vi "Read Measure--SubVI.vi"(8 "error in (no error)":errorcluster, 10 "Device":T9, 11 "Data Cluster":T1 {"Flexi-Flow Devices"."Control State"."Control Mode" items=["Bus/RS232"=0, "FLOW-BUS slave"=2, "Valve close"=3, "Controller idle"=4, "Setpoint 100%"=7, "Valve fully open"=8, "Calibration mode"=9, "Setpoint 0%"=12, "RS232"=18, "Valve steering"=20, "Valve safe state"=22]}) -> (0 "error out":errorcluster, 3 "Data Cluster Out":T1 {"Flexi-Flow Devices"."Control State"."Control Mode" items=["Bus/RS232"=0, "FLOW-BUS slave"=2, "Valve close"=3, "Controller idle"=4, "Setpoint 100%"=7, "Valve fully open"=8, "Calibration mode"=9, "Setpoint 0%"=12, "RS232"=18, "Valve steering"=20, "Valve safe state"=22]})   [LabVIEW 2024, in "FlexiFlowInterfaceCH2.lvlib"]
uses:
  FlexiFlowInterfaceCH2.lvlib
  FlexiFlowDevice--enum.ctl
  Module Data--cluster.ctl
  Modbus TCP Connection Settings--cluster.ctl
  Modbus Flexi-Flow State--cluster.ctl
  <vilib>/Plasmionique/MB Master/MB_Master_TCP/MB_Master_TCP.lvclass
  Device Type--enum.ctl
  Modbus Flexi-Flow Controls--cluster.ctl
  Modbus Flexi-Flow API/Control Mode--enum.ctl
  Modbus Flexi-Flow API/Control Function Values--enum.ctl
  Modbus Flexi-Flow Measure State--cluster.ctl
  Modbus Flexi-Flow API/Bronkhorst Flexi-Flow ModbusTCP API.lvlib
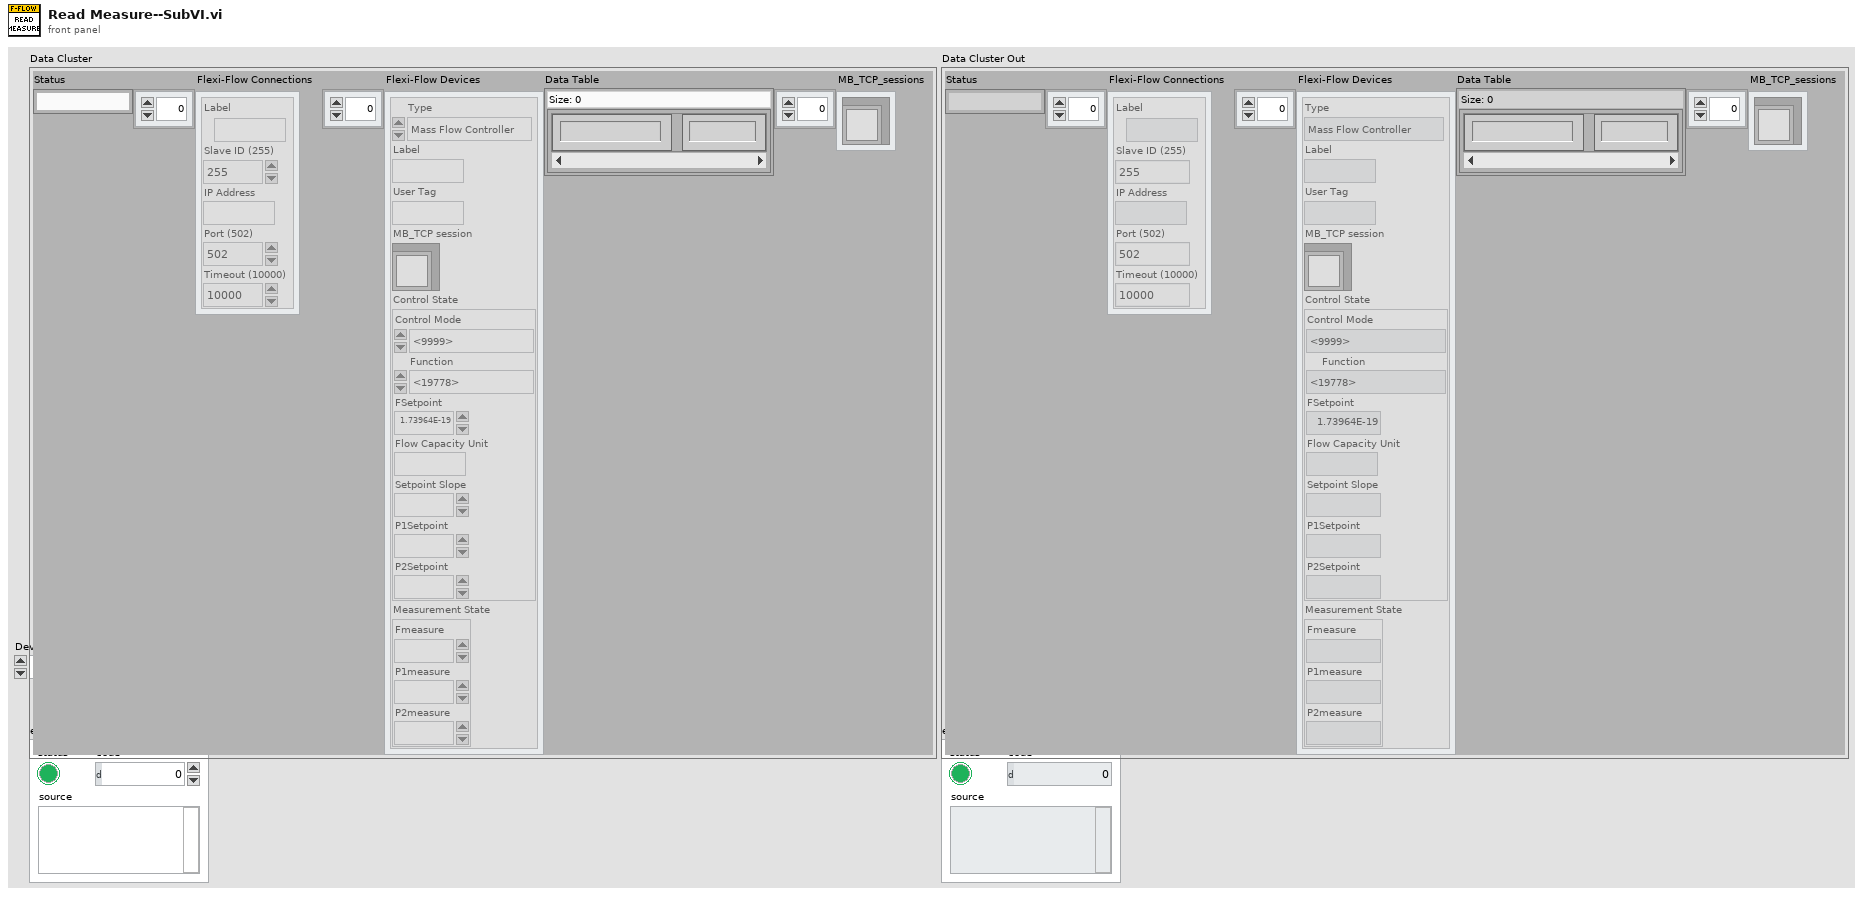
[diagram p1: front panel]
types:
  T1 = typedef "FlexiFlowInterfaceCH2.lvlib/Module Data--cluster.ctl" = cluster{"Status":string, "Flexi-Flow Connections":T2[], "Flexi-Flow Devices":T3[], "Data Table":map{string, dbl}, "MB_TCP_sessions":refnum<class "MB_Master_TCP.lvclass">[]}
  T2 = typedef "FlexiFlowInterfaceCH2.lvlib/Modbus TCP Connection Settings--cluster.ctl" = cluster{"Label":string, "Slave ID (255)":u8, "IP Address":string, "Port (502)":u16, "Timeout (10000)":i32}
  T3 = typedef "FlexiFlowInterfaceCH2.lvlib/Modbus Flexi-Flow State--cluster.ctl" = cluster{"Type":T4, "Label":string, "User Tag":string, "MB_TCP session":refnum<class "MB_Master_TCP.lvclass">, "Control State":T5, "Measurement State":T8}
  T4 = typedef "FlexiFlowInterfaceCH2.lvlib/Device Type--enum.ctl" = enum16{"Mass Flow Controller", "Mass Flow Meter"}
  T5 = typedef "FlexiFlowInterfaceCH2.lvlib/Modbus Flexi-Flow Controls--cluster.ctl" = cluster{"Control Mode":T6, "Function":T7, "FSetpoint":sgl, "Flow Capacity Unit":string, "Setpoint Slope":u16, "P1Setpoint":sgl, "P2Setpoint":sgl}
  T6 = typedef "Bronkhorst Flexi-Flow ModbusTCP API.lvlib/Control Mode--enum.ctl" = u16
  T7 = typedef "Bronkhorst Flexi-Flow ModbusTCP API.lvlib/Control Function Values--enum.ctl" = enum16{"Flow", "Upstream pressure", "Downstream pressure", "Flow with upstream pressure limit", "Flow with downstream pressure limit", "Upstream pressure with flow limit", "Downstream pressure with flow limit"}
  T8 = typedef "FlexiFlowInterfaceCH2.lvlib/Modbus Flexi-Flow Measure State--cluster.ctl" = cluster{"Fmeasure":dbl, "P1measure":sgl, "P2measure":sgl}
  T9 = typedef "FlexiFlowInterfaceCH2.lvlib/FlexiFlowDevice--enum.ctl" = enum16{"Hydrogen Inlet", "Nitrogen Inlet", "Cathode Outlet", "Anode Outlet"}
  T10 = typedef "Bronkhorst Flexi-Flow ModbusTCP API.lvlib/Fmeasure (F,P1,P2)--cluster.ctl" = cluster{"Fmeasure (F)":sgl, "Fmeasure (P1)":sgl, "Fmeasure (P2)":sgl}
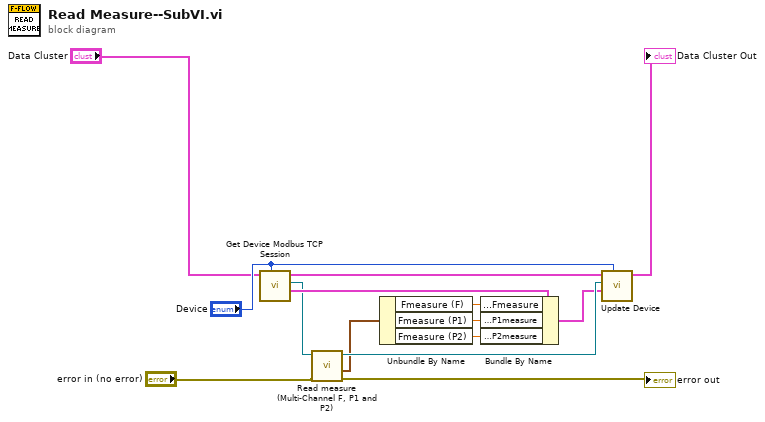
[diagram p0: block diagram]
diagram:
  n1 = call "Get Device Modbus TCP Session.vi"("Device"="Device", "Data Cluster In"="Data Cluster") -> ("Device State"=w11:T3, "MB_TCP session"=w10:refnum<class "MB_Master_TCP.lvclass">, "Data Cluster Out"=w1:T1)  [unwired: 7 in]
  n2 = call "Read measure (Multi-Channel F, P1 and P2).vi"("error in"="error in (no error)", "MB_TCP session in"=w10) -> ("error out"=→"error out":errorcluster, "Fmeasure (F, P1, P2)"=w6:T10, "MB session out"=w13:refnum<class "MB_Master_TCP.lvclass">)  [unwired: 7 in]
  n3 = Unbundle By Name(w6) -> ("Fmeasure (F)"=w7:sgl, "Fmeasure (P1)"=w9:sgl, "Fmeasure (P2)"=w8:sgl)
  n4 = Bundle By Name(cluster=w11, "Measurement State.Fmeasure"=w7, "Measurement State.P1measure"=w9, "Measurement State.P2measure"=w8) -> (w12:T3)
  n5 = call "Update Device.vi"("Device"="Device", "Device State"=w12, "MB_TCP session"=w13, "Data Cluster"=w1) -> ("Data Cluster Out"=→"Data Cluster Out":T1)  [unwired: 7 in]
